vi "Example - Set configuration.vi"() -> ()   [LabVIEW 2016, in "Mercury iXX.lvlib"]
uses:
  Mercury iXX.lvlib
  Public/Libraries/Temperature/Controls/Temperature Device (Read).ctl
  Public/Controls/Manufacturing Data.ctl
  Public/Libraries/Temperature/Controls/Temperature Sensor Type.ctl
  Public/Libraries/Temperature/Controls/Excitation Cluster.ctl
  Public/Libraries/Temperature/Controls/Excitation Type.ctl
  Public/Libraries/Temperature/Controls/Calibration Cluster.ctl
  Public/Libraries/Temperature/Controls/Calibration Interpolation.ctl
  Public/Libraries/Temperature/Controls/Loop Cluster.ctl
  Public/Libraries/Temperature/Controls/Temperature Signals Cluster.ctl
  Public/Libraries/Heater/Controls/Heater Device (Read).ctl
  Public/Libraries/Heater/Controls/Heater Signals Cluster.ctl
  Public/Libraries/Temperature/Controls/Temperature Device (Set).ctl
  Public/Libraries/Heater/Controls/Heater Device (Set).ctl
  Public/Controls/Comms Transport Layer.ctl
  Public/Controls/ISOBus Address.ctl
  Private/Controls/Lookup Reference FGV Enum.ctl
  Public/Libraries/System/Open/Open System.vi
  Public/Libraries/System/Read/Catalogue (Read).vi
  Public/Libraries/System/Open/Open Device.vi
  Public/Libraries/System/Set/Date (Set).vi
  Public/Libraries/System/Read/DateTime (Read).vi
  Public/Libraries/Temperature/Configuration/Set/Temperature Device (Set).vi
  Public/Libraries/Temperature/Configuration/Read/Temperature Device (Read).vi
  Public/Libraries/Heater/Configuration/Set/Heater Device (Set).vi
  Public/Libraries/Heater/Configuration/Read/Heater Device (Read).vi
  Public/Libraries/System.lvlib
  Public/Libraries/System/Set/Time (Set).vi
  Public/Libraries/Temperature.lvlib
  Public/Libraries/Heater.lvlib
panel:
  out "time stamp":timestamp
  in  "Heater Device Settings":T1
  in  "Temperature Device Settings":T3
  out "Heater Device Settings Read":T10
  out "Temperature Device Settings read":T12
  out "Devices":string[](array[string])
  out "Set Date Response":string
  out "Set Time Response":string
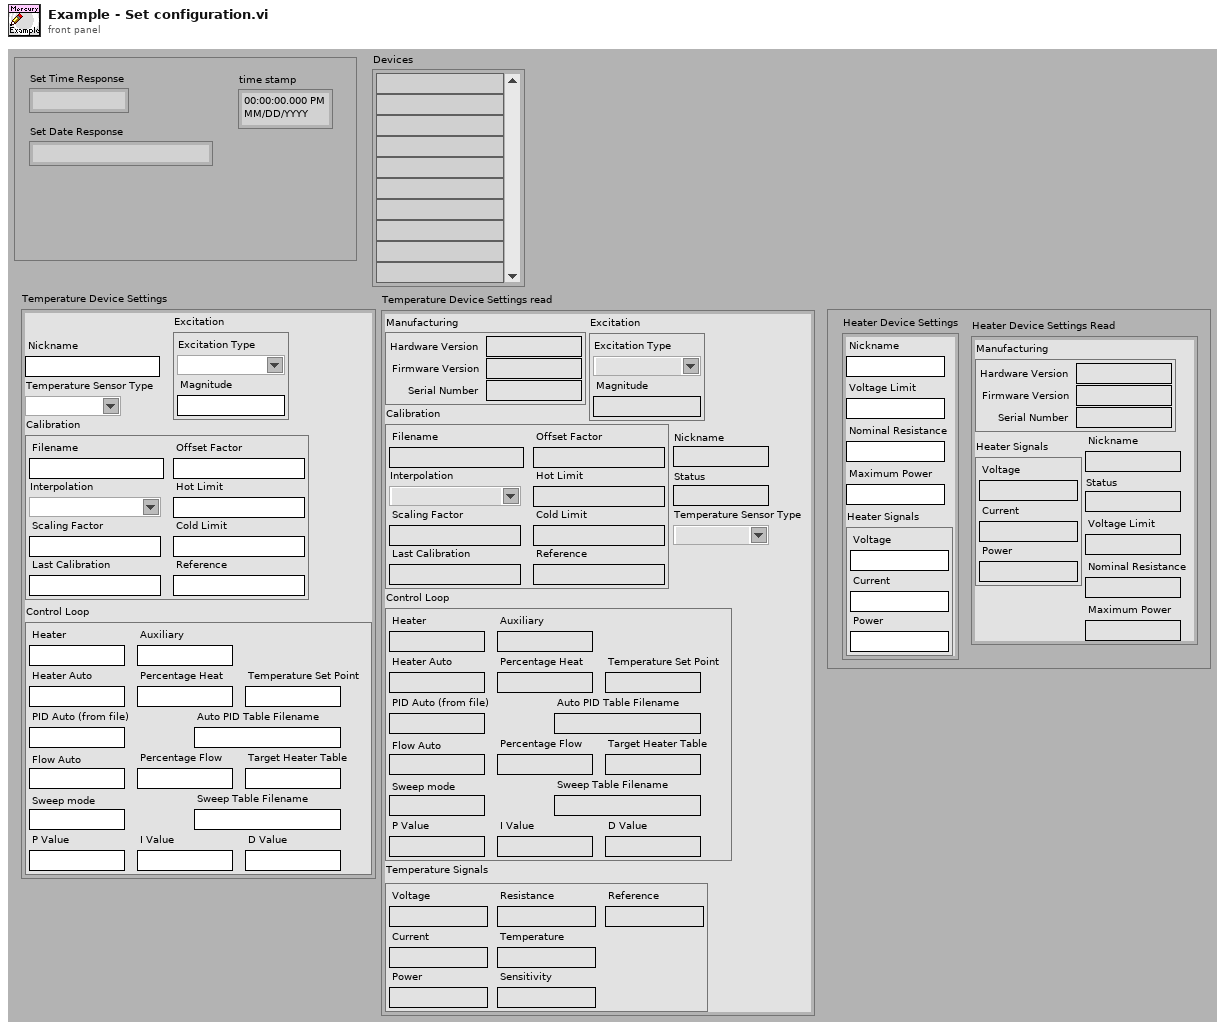
[diagram p1: front panel]
types:
  T1 = typedef "Mercury iXX.lvlib/Heater.lvlib/Heater Device (Set).ctl" = cluster{"Nickname":string, "Voltage Limit":string, "Nominal Resistance":string, "Maximum Power":string, "Heater Signals":T2}
  T2 = typedef "Mercury iXX.lvlib/Heater.lvlib/Heater Signals Cluster.ctl" = cluster{"Voltage":string, "Current":string, "Power":string}
  T3 = typedef "Mercury iXX.lvlib/Temperature.lvlib/Temperature Device (Set).ctl" = cluster{"Nickname":string, "Temperature Sensor Type":T4, "Excitation":T5, "Calibration":T7, "Control Loop":T9}
  T4 = typedef "Mercury iXX.lvlib/Temperature.lvlib/Temperature Sensor Type.ctl" = string
  T5 = typedef "Mercury iXX.lvlib/Temperature.lvlib/Excitation Cluster.ctl" = cluster{"Excitation Type":T6, "Magnitude":string}
  T6 = typedef "Mercury iXX.lvlib/Temperature.lvlib/Excitation Type.ctl" = string
  T7 = typedef "Mercury iXX.lvlib/Temperature.lvlib/Calibration Cluster.ctl" = cluster{"Filename":string, "Interpolation":T8, "Scaling Factor":string, "Offset Factor":string, "Hot Limit":string, "Cold Limit":string, "Last Calibration":string, "Reference":string}
  T8 = typedef "Mercury iXX.lvlib/Temperature.lvlib/Calibration Interpolation.ctl" = string
  T9 = typedef "Mercury iXX.lvlib/Temperature.lvlib/Loop Cluster.ctl" = cluster{"Heater":string, "Auxiliary":string, "Heater Auto":string, "Percentage Heat":string, "Temperature Set Point":string, "PID Auto (from file)":string, "P Value":string, "I Value":string, "D Value":string, "Auto PID Table Filename":string, "Flow Auto":string, "Target Heater Table":string, "Sweep mode":string, "Sweep Table Filename":string, "Percentage Flow":string}
  T10 = typedef "Mercury iXX.lvlib/Heater.lvlib/Heater Device (Read).ctl" = cluster{"Manufacturing":T11, "Nickname":string, "Voltage Limit":string, "Nominal Resistance":string, "Maximum Power":string, "Heater Signals":T2, "Status":string}
  T11 = typedef "Mercury iXX.lvlib/Manufacturing Data.ctl" = cluster{"Hardware Version":string, "Firmware Version":string, "Serial Number":string}
  T12 = typedef "Mercury iXX.lvlib/Temperature.lvlib/Temperature Device (Read).ctl" = cluster{"Manufacturing":T11, "Temperature Sensor Type":T4, "Excitation":T5, "Calibration":T7, "Control Loop":T9, "Temperature Signals":T13, "Nickname":string, "Status":string}
  T13 = typedef "Mercury iXX.lvlib/Temperature.lvlib/Temperature Signals Cluster.ctl" = cluster{"Voltage":string, "Current":string, "Power":string, "Resistance":string, "Temperature":string, "Sensitivity":string, "Reference":string}
  T14 = typedef "Mercury iXX.lvlib/ISOBus Address.ctl" = i32
  T15 = typedef "Mercury iXX.lvlib/Comms Transport Layer.ctl" = enum16{"Ethernet TCP/IP", "USB", "ISOBus - RS-232", "GPIB"}
  T16 = typedef "Mercury iXX.lvlib/Mercury Reference.ctl" = cluster{"Comms":refnum<visa-resource-name>, "Device ID":string[], "Comms Layer":T15, "Command":string, "Query reference":T17}
  T17 = typedef "Mercury iXX.lvlib/Query Dynamic Reference.ctl" = refnum<vi>
  T18 = typedef "Mercury iXX.lvlib/Response String.ctl" = string
  T19 = typedef "Mercury iXX.lvlib/Lookup Reference FGV Enum.ctl" = enum16{"Check VISA", "Get VI Ref", "Set VI ref", "Delete Single Ref", "Clear All"}
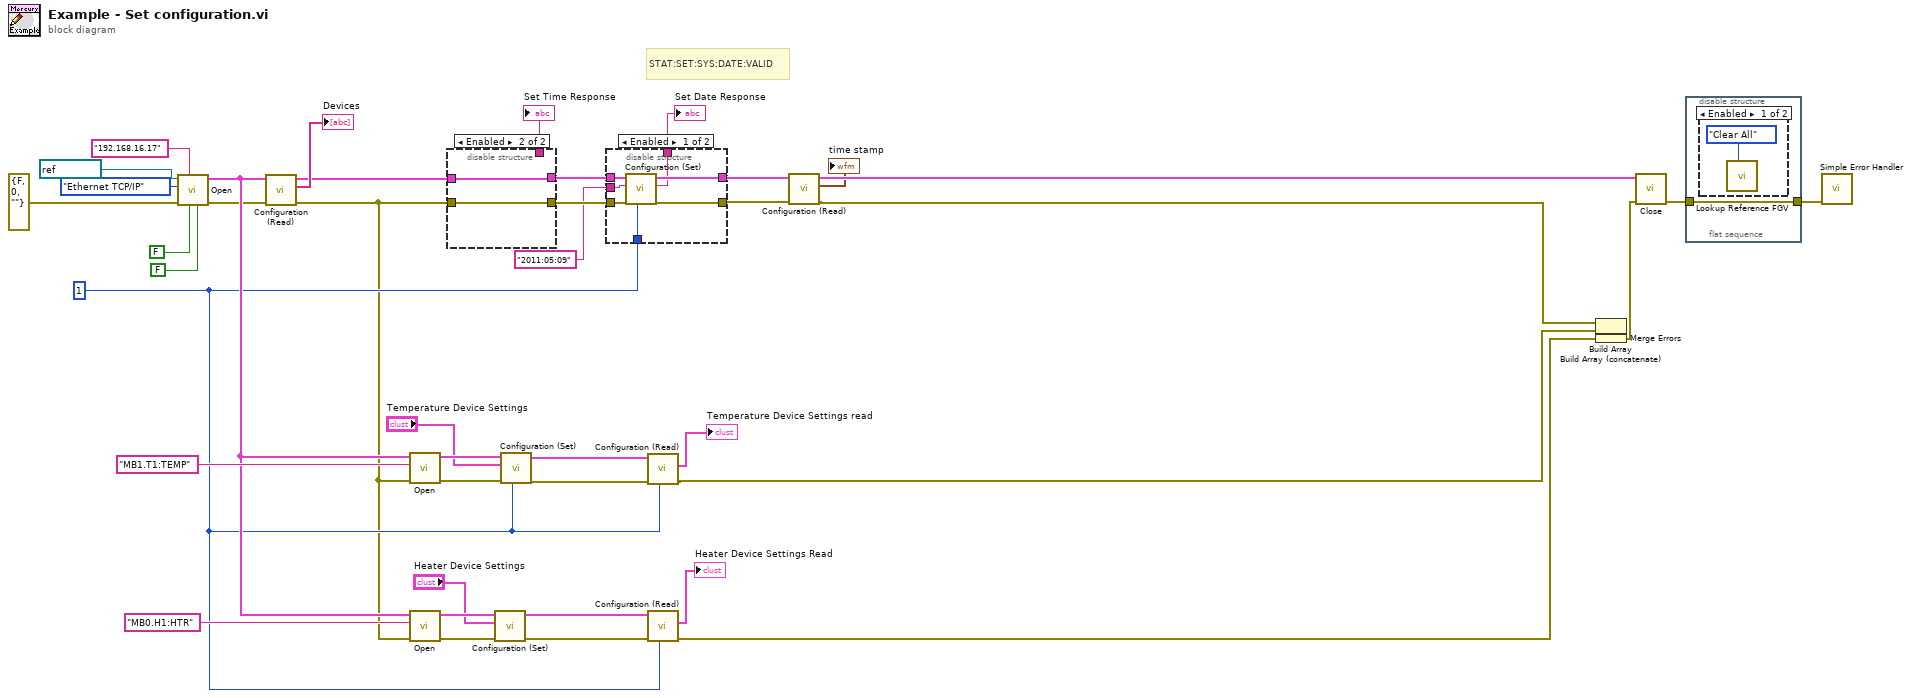
[diagram p0: block diagram]
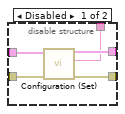
[diagram p4: hidden frame]
diagram:
  w11 = T14 1 ("ISOBUS address")
  # "STAT:SET:SYS:DATE:VALID"
  n1 = call-poly "Open.vi"("Clear Previous Connections (False)"=FALSE ("Reset (True)"), "ID Query (True)"=FALSE, "IP Address"="192.168.16.17", "error in (no error)"=errorcluster {"status"=FALSE, "code"=0, "source"=""}, "Comms Layer"=Comms_Transport_Layer."Ethernet TCP/IP", "VISA resource name"=refnum<visa-resource-name> "COM1") -> ("error out"=w27:errorcluster, "Mercury Reference Out"=w28:T16)  [unwired: 1 in, 3 out]
  n2 = call-poly "Configuration (Read).vi"("error in"=w27, "Mercury Reference In"=w28) -> ("error out"=w5:errorcluster, "Devices"=→"Devices":string[], "Mercury Reference Out"=w25:T16)  [unwired: 1 in, 6 out]
  n3 = call-poly "Open.vi"("error in (no error)"=w5, "Device Identifier"="MB1.T1:TEMP", "Mercury Reference In"=w28) -> ("error out"=w24:errorcluster, "Mercury Reference Out"=w23:T16)  [unwired: 1 in, 6 out]
  n4 = call-poly "Open.vi"("error in (no error)"=w5, "Device Identifier"="MB0.H1:HTR", "Mercury Reference In"=w28) -> ("error out"=w16:errorcluster, "Mercury Reference Out"=w15:T16)  [unwired: 1 in, 6 out]
  n5 = disable-structure shown="Enabled" {
    disable-tunnel: w25 -> [w48 w50]
    disable-tunnel: w5 -> [w47 w49]
    disable-tunnel: [w46 w49] -> w40
    disable-tunnel: [w45 w50] -> w39
    disable-tunnel: [w44 _] -> w38
    frame Disabled {
      n6 = call-poly "Configuration (Set).vi"("error in"=w47, "Mercury Reference In"=w48) -> ("error out"=w46:errorcluster, "Response"=w44:T18, "Mercury Reference Out"=w45:T16)  [unwired: 6 in, 1 out]
    }
    frame Enabled {
    }
  }
  "Set Time Response" <- w38
  n7 = call-poly "Configuration (Set).vi"("error in"=w16, "Heater Device Settings"="Heater Device Settings", "Mercury Reference In"=w15) -> ("error out"=w14:errorcluster, "Mercury Reference Out"=w13:T16)  [unwired: 1 in, 6 out]
  n8 = call-poly "Configuration (Set).vi"("ISOBUS address"=w11, "error in"=w24, "Temperature Device Settings"="Temperature Device Settings", "Mercury Reference In"=w23) -> ("error out"=w19:errorcluster, "Mercury Reference Out"=w18:T16)  [unwired: 6 out]
  n9 = disable-structure shown="Enabled" {
    disable-tunnel: w40 -> [w57 w58]
    disable-tunnel: w39 -> [w56 w59]
    disable-tunnel: [w55 w59] -> w8
    disable-tunnel: [w54 w58] -> w7
    disable-tunnel: [w53 _] -> w37
    disable-tunnel: "2011:05:09" ("Date") -> [w52 _]
    disable-tunnel: w11 -> [w51 _]
    frame Enabled {
      n10 = call-poly "Configuration (Set).vi"("ISOBUS address"=w51, "error in"=w57, "Date"=w52, "Mercury Reference In"=w56) -> ("error out"=w54:errorcluster, "Response"=w53:T18, "Mercury Reference Out"=w55:T16)  [unwired: 5 out]
    }
    frame Disabled {
    }
  }
  "Set Date Response" <- w37
  n11 = call-poly "Configuration (Read).vi"("ISOBUS address"=w11, "error in"=w19, "Mercury Reference In"=w18) -> ("error out"=w20:errorcluster, "Device Details"=→"Temperature Device Settings read":T12)  [unwired: 7 out]
  n12 = call-poly "Configuration (Read).vi"("ISOBUS address"=w11, "error in"=w14, "Mercury Reference In"=w13) -> ("error out"=w22:errorcluster, "Device Details"=→"Heater Device Settings Read":T10)  [unwired: 7 out]
  n13 = call-poly "Configuration (Read).vi"("error in"=w7, "Mercury Reference In"=w8) -> ("error out"=w9:errorcluster, "time stamp"=→"time stamp":timestamp, "Mercury Reference Out"=w10:T16)  [unwired: 1 in, 6 out]
  n14 = Build Array(w9, w20, w22) -> (w2:errorcluster[])
  n15 = Build Array (concatenate)(w2) -> (w1:errorcluster[])
  n16 = Merge Errors(w1) -> (w32:errorcluster)
  n17 = call "Close.vi"("error in (no error)"=w32, "Mercury Reference"=w10) -> ("error out"=w30:errorcluster)  [unwired: 9 out]
  n18 = flat-sequence {
    tunnel: [w60] -> w31
    tunnel: w30 -> [w60]
    frame #0 {
      n19 = disable-structure shown="Enabled" {
        frame Enabled {
          n20 = call "Lookup Reference FGV.vi"("State"=Lookup_Reference_FGV_Enum."Clear All") -> ()  [unwired: 4 in, 7 out]
        }
        frame Disabled {
        }
      }
    }
  }
  n21 = call <vilib>:"Simple Error Handler.vi"("error in (no error)"=w31) -> ()  [unwired: 1 in, 8 out]
